vi "Update Channel Name Status.vi"(8 "error in (no error)":errorcluster, 10 "Ctl Reference":T3, 11 "Display State In":T1) -> (0 "error out":errorcluster, 1 "Data":u16, 2 "Ctl Reference Out":T3, 3 "Display StateOut":T1)   [LabVIEW 2021, in "myRIO Channel Name.xctl"]
uses:
  <vilib>/myRIO/Common/Express VI Framework/xctls/myRIO Channel Name/myRIO Channel Name.xctl
  <vilib>/myRIO/Common/Express VI Framework/xctls/myRIO Channel Name/State.ctl
  <vilib>/myRIO/Common/Express VI Framework/typedefs/Data Validate Ref.ctl
  <vilib>/myRIO/Common/Express VI Framework/vis/Express VI Framework Strings Global.vi
  <vilib>/regexp/Match Regular Expression.xnode
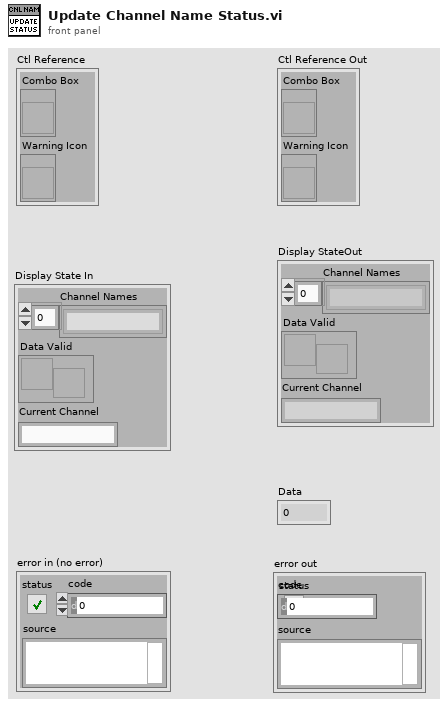
[diagram p1: front panel]
types:
  T1 = typedef "myRIO Channel Name.xctl/State.ctl" = cluster{"Channel Names":string[], "Data Valid":T2, "Current Channel":string}
  T2 = typedef "Data Validate Ref.ctl" = refnum<user-event>
  T3 = cluster{"Combo Box":refnum<vi>, "Warning Icon":refnum<vi>}
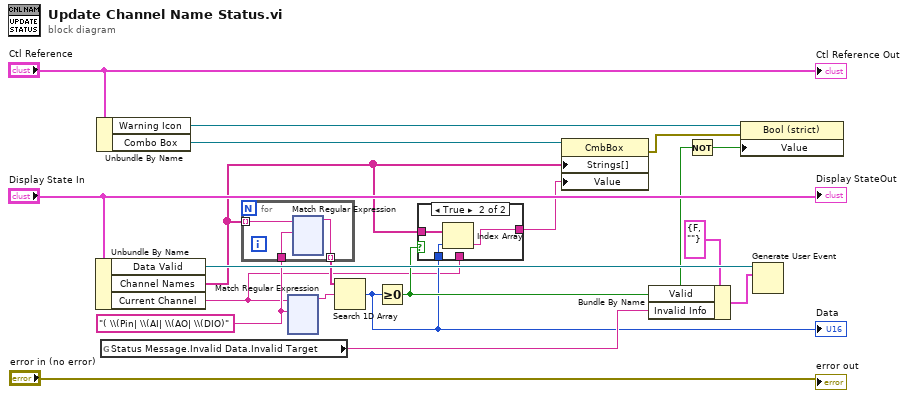
[diagram p0: block diagram]
diagram:
  w7 = "( \\(Pin| \\(AI| \\(AO| \\(DIO)" ("regular expression")
  n1 = Unbundle By Name("Display State In") -> ("Data Valid"=w13:T2, "Channel Names"=w4:string[], "Current Channel"=w2:string)
  n2 = Unbundle By Name("Ctl Reference") -> ("Warning Icon"=w18:refnum<vi>, "Combo Box"=w16:refnum<vi>)
  n3 = global read "Express VI Framework Strings Global.vi" "Status Message.Invalid Data.Invalid Target"() -> (w9:string)
  n4 = for {
    tunnel: w4 -> [w22] mode=indexing
    tunnel: w7 -> [w21]
    tunnel: [w20] -> w6 mode=indexing
    n5 = xnode "Match Regular Expression"("input string"=w22, "regular expression"=w21) -> ("before match"=w20:string)  [unwired: 4 in, 4 out]
  }
  n6 = xnode "Match Regular Expression"("input string"=w2, "regular expression"=w7) -> ("before match"=w8:string)  [unwired: 4 in, 4 out]
  n7 = Search 1D Array(1D array=w6, element=w8) -> (index of element=w3:i32)  [unwired: 1 in]
  "Data" <- w3
  n8 = Greater Or Equal To 0?(x=w3) -> (x >= 0?=w5:bool)
  n9 = case shown="True" w5 {
    tunnel: w4 -> [_ w143]
    tunnel: w3 -> [_ w142]
    tunnel: w2 -> [w140 _]
    tunnel: [w140 w141] -> w1
    frame False {
    }
    frame True {
      n10 = Index Array(array=w143, index=w142) -> (element=w141:string)
    }
  }
  n11 = property class="CmbBox"(reference=w16, "Strings[]"=w4, "Value"=w1) -> (error out=w17:errorcluster)  [unwired: 1 in, 1 out]
  n12 = Bundle By Name(cluster=cluster{"Valid":bool, "Invalid Info":string} {"Valid"=FALSE, "Invalid Info"=""} ("event data"), "Valid"=w5, "Invalid Info"=w9) -> (w10:cluster{"Valid":bool, "Invalid Info":string})
  n13 = Not(x=w5) -> (.not. x?=w14:bool)
  n14 = property class="Bool (strict)"(reference=w18, error in=w17, "Value"=w14) -> ()  [unwired: 2 out]
  n15 = Generate User Event(user event=w13, event data cluster=w10) -> ()  [unwired: 2 in, 2 out]
  "error out" <- "error in (no error)"
  "Ctl Reference Out" <- "Ctl Reference"
  "Display StateOut" <- "Display State In"
